vi "string-unbundler-4.vi"(0 "String":string) -> (1 "Array 1":dbl[](array[numeric]), 2 "Array 2":dbl[](array[numeric]), 3 "Array 3":dbl[](array[numeric]), 4 "Array 4":dbl[](array[numeric]))   [LabVIEW 2023]
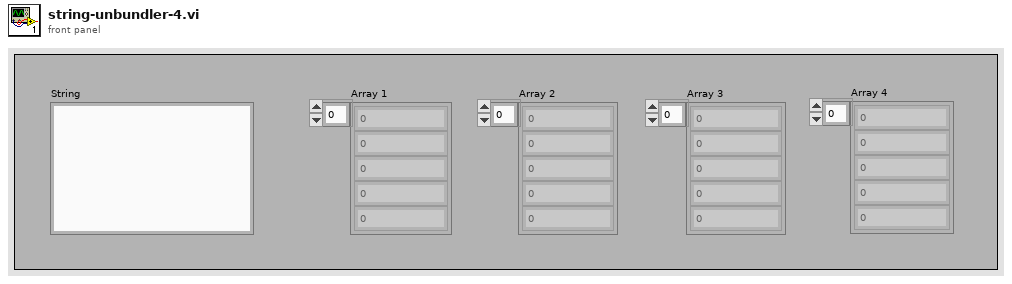
[diagram p1: front panel]
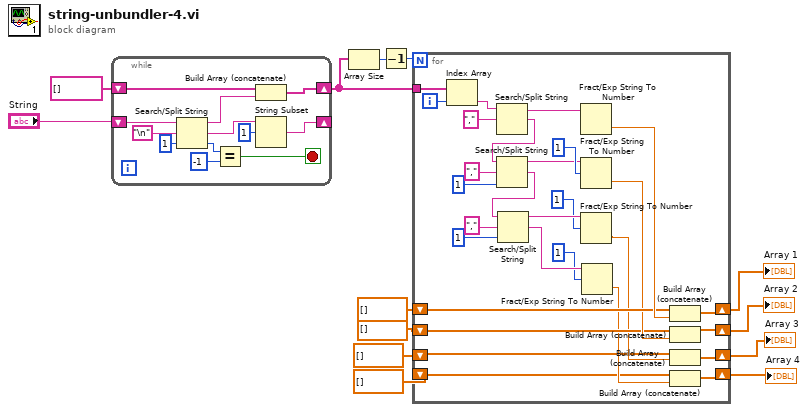
[diagram p0: block diagram]
diagram:
  n1 = while {
    shift-right: [w22] -> w13
    shift-left: string[] [] -> [w24]
    shift-right: [w16] -> _
    shift-left: "String" -> [w23]
    stop <- w19 stop-if-true
    n2 = Search/Split String(string=w23, search string/char (-)="\n", offset (0)=1) -> (substring before match=w25:string, match + rest of string=w17:string, offset of match=w21:i32)
    n3 = Equal?(x=w21, y=-1) -> (x = y?=w19:bool)
    n4 = Build Array (concatenate)(w24, w25) -> (w22:string[])
    n5 = String Subset(string=w17, offset (0)=1) -> (substring=w16:string)  [unwired: 1 in]
  }
  n6 = Array Size(array=w13) -> (size(s)=w7:i32)
  n7 = Decrement(x=w7) -> (x-1=w8:i32)
  n8 = for {
    N: w8 -> [_]
    tunnel: w13 -> [w54]
    shift-right: [w44] -> w3
    shift-left: dbl[] [] -> [w47]
    shift-right: [w49] -> w4
    shift-left: dbl[] [] -> [w45]
    shift-right: [w29] -> w5
    shift-left: dbl[] [] -> [w31]
    shift-right: [w28] -> w6
    shift-left: dbl[] [] -> [w30]
    i -> [w53]
    n9 = Index Array(array=w54, index=w53) -> (element=w52:string)
    n10 = Search/Split String(string=w52, search string/char (-)=",") -> (substring before match=w50:string, match + rest of string=w40:string)  [unwired: 1 in, 1 out]
    n11 = Search/Split String(string=w40, search string/char (-)=",", offset (0)=1) -> (substring before match=w38:string, match + rest of string=w39:string)  [unwired: 1 out]
    n12 = Search/Split String(string=w39, search string/char (-)=",", offset (0)=1) -> (substring before match=w35:string, match + rest of string=w37:string)  [unwired: 1 out]
    n13 = Fract/Exp String To Number(string=w50) -> (number=w48:dbl)  [unwired: 3 in, 1 out]
    n14 = Fract/Exp String To Number(string=w38, offset=1) -> (number=w46:dbl)  [unwired: 2 in, 1 out]
    n15 = Fract/Exp String To Number(string=w35, offset=1) -> (number=w33:dbl)  [unwired: 2 in, 1 out]
    n16 = Fract/Exp String To Number(string=w37, offset=1) -> (number=w32:dbl)  [unwired: 2 in, 1 out]
    n17 = Build Array (concatenate)(w47, w48) -> (w44:dbl[])
    n18 = Build Array (concatenate)(w45, w46) -> (w49:dbl[])
    n19 = Build Array (concatenate)(w31, w33) -> (w29:dbl[])
    n20 = Build Array (concatenate)(w30, w32) -> (w28:dbl[])
  }
  "Array 1" <- w3
  "Array 2" <- w4
  "Array 3" <- w5
  "Array 4" <- w6
